vi "Phasor Explorer Zero Finder tau (Discrete, Gated Phasor).vi"(4 "data":variant, 5 "x":dbl) -> (2 "f(x)":dbl)   [LabVIEW 2021, in "Phasor Explorer.lvlib"]
uses:
  Phasor tau_phi & tau_m Zero Finder Parameters.ctl
  Phasor Explorer.lvlib
  Phasor.lvlib
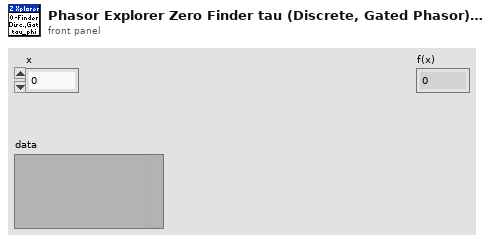
[diagram p1: front panel]
types:
  T1 = typedef "Phasor.lvlib/Phasor tau_phi & tau_m Zero Finder Parameters.ctl" = cluster{"Period":ext, "Width":ext, "# Gates":ext, "f":ext, "tan(phi), m":ext, "phi(T)/m(F)":bool, "Offset":ext}
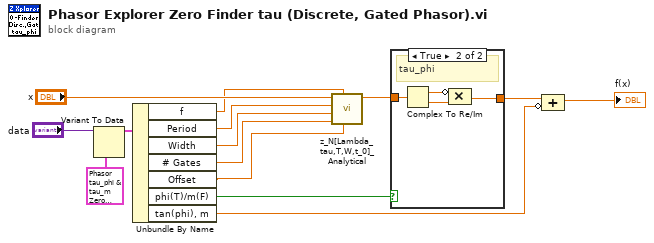
[diagram p0: block diagram]
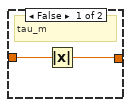
[diagram p2: hidden frame]
diagram:
  n1 = Variant To Data(type=T1 {"Period"=0.0, "Width"=0.0, "# Gates"=0.0, "f"=0.0, "tan(phi), m"=0.0, "phi(T)/m(F)"=TRUE, "Offset"=0.0} ("cluster"), Variant="data") -> (data=w3:T1)  [unwired: 1 in, 1 out]
  n2 = Unbundle By Name(w3) -> ("f"=w4:ext, "Period"=w11:ext, "Width"=w10:ext, "# Gates"=w9:ext, "Offset"=w2:ext, "phi(T)/m(F)"=w7:bool, "tan(phi), m"=w1:ext)
  n3 = call "z_N[Lambda_tau,T,W,t_0]_Analytical.vi"("t0"=w2, "Harmonic f"=w4, "N"=w9, "W"=w10, "T"=w11, "tau"="x") -> ("z_n,N,W(tau)"=w14:cxt)  [unwired: 5 in]
  n4 = case shown="True" w7 {
    tunnel: w14 -> [w16 w20]
    tunnel: [w15 w17] -> w6
    frame False {
      # "tau_m"
      n5 = Absolute Value(x=w16) -> (abs(x)=w15:ext)
    }
    frame True {
      # "tau_phi"
      n6 = Complex To Re/Im(x + iy=w20) -> (x=w19:ext, y=w18:ext)
      n7 = Compound Arithmetic op=MULTIPLY(invert w19, w18) -> (w17:ext)
    }
  }
  n8 = Compound Arithmetic op=ADD(w6, invert w1) -> (→"f(x)":ext)
